vi "Start.vi"(8 "error in":errorcluster, 11 "CAN Task in":refnum<class "CANopen Task Actor.lvclass">) -> (0 "error out":errorcluster, 3 "CAN Task out":refnum<class "CANopen Task Actor.lvclass">)   [LabVIEW 2024, in "CANopen Task Actor.lvlib" / "CANopen Task Actor.lvclass"]
uses:
  CANopen Task Actor.lvclass
  CANopen Task Actor.lvclass/CANopen Task Actor.ctl
  <vilib>/ActorFramework/Actor/Actor.lvclass
  CAN Task Messages/Do Msg/Do Msg.lvclass
  C:/Program Files/National Instruments/LabVIEW 2024/vi.lib/ActorFramework/Message/Message.lvclass
  D:/git/CANopen-XNET/CANopen/CAN Task/CAN Task Messages/Do Msg/Do Msg.lvclass
  C:/Program Files/National Instruments/LabVIEW 2024/vi.lib/ActorFramework/Actor/Actor.lvclass
  D:/git/CANopen-XNET/CANopen/CAN Task/CAN Task/CANopen Task Actor.lvclass
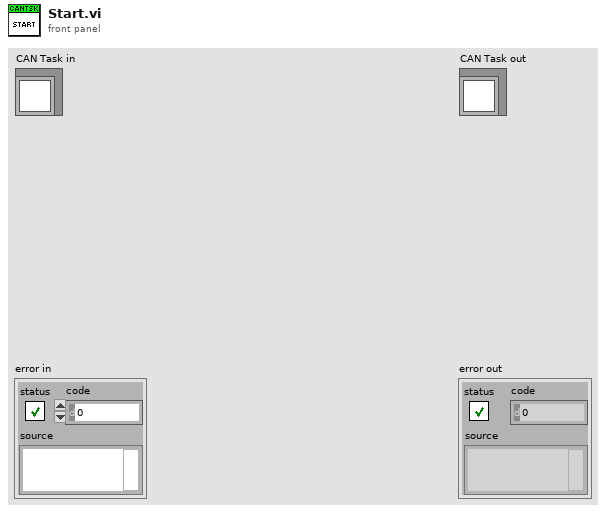
[diagram p1: front panel]
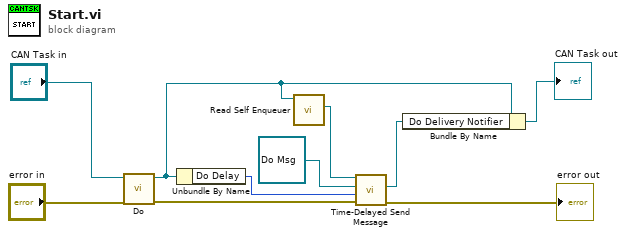
[diagram p0: block diagram]
diagram:
  n1 = call "Do.vi"("error in"="error in", "CAN Task in"="CAN Task in") -> ("error out"=w3:errorcluster, "CAN Task out"=w1:refnum<class "CANopen Task Actor.lvclass">)  [unwired: 8 in]
  n2 = Unbundle By Name(w1) -> ("Do Delay"=w7:i32)
  n3 = call <vilib>:"Read Self Enqueuer.vi"("Actor"=w1) -> ("Self Enqueuer"=w9:refnum<class "Message Enqueuer.lvclass">)  [unwired: 10 in]
  n4 = call <vilib>:"Time-Delayed Send Message.vi"("error in (no error)"=w3, "Milliseconds To Wait"=w7, "Message"=refnum<class "Do Msg.lvclass"> refnum ("CANopen.lvlib:CAN Task.lvlib:Do Msg.lvclass"), "Message Enqueuer"=w9) -> ("error out"=→"error out":errorcluster, "Delivery Notifier"=w5:refnum<notifier>)  [unwired: 6 in]
  n5 = Bundle By Name(cluster=w1, "Do Delivery Notifier"=w5) -> (→"CAN Task out":refnum<class "CANopen Task Actor.lvclass">)
